vi "Vision Tracking Drive Control.vi"(11 "Cluster In":T11) -> (3 "Cluster Out":T11)   [LabVIEW 2018]
uses:
  <vilib>/Rock Robotics/WPI/MotorControl/WPI_MotorControlDeviceRef.ctl
  <vilib>/Rock Robotics/WPI/MotorControl/WPI_MotorControlType.ctl
  <vilib>/Rock Robotics/SystemInterfaces/DIO/FPGA_DIOPWMChannel.ctl
  <vilib>/Rock Robotics/WPI/PWM/WPI_PWMDeadband.ctl
  <vilib>/Rock Robotics/SystemInterfaces/DIO/FPGA_DIOChannel.ctl
  <vilib>/Rock Robotics/WPI/Joystick/WPI_JoystickDevRef.ctl
  <vilib>/Rock Robotics/WPI/Joystick/WPI_JoystickDeviceEnum.ctl
  <vilib>/Rock Robotics/WPI/DriverStation/WPI_DriverStationRobotMode2.ctl
  <vilib>/Rock Robotics/WPI/RobotDrive/WPI_RobotDriveDevRef.ctl
  Vision States.ctl
  <vilib>/Rock Robotics/WPI/ThirdParty/Phoenix-LabVIEW/Motor Controller/Controls/CTRE_Phoenix_MotorControl_ControlMode.ctl
  <vilib>/Rock Robotics/Network Tables/NT Read Number.vi
  Robot Global Data.vi
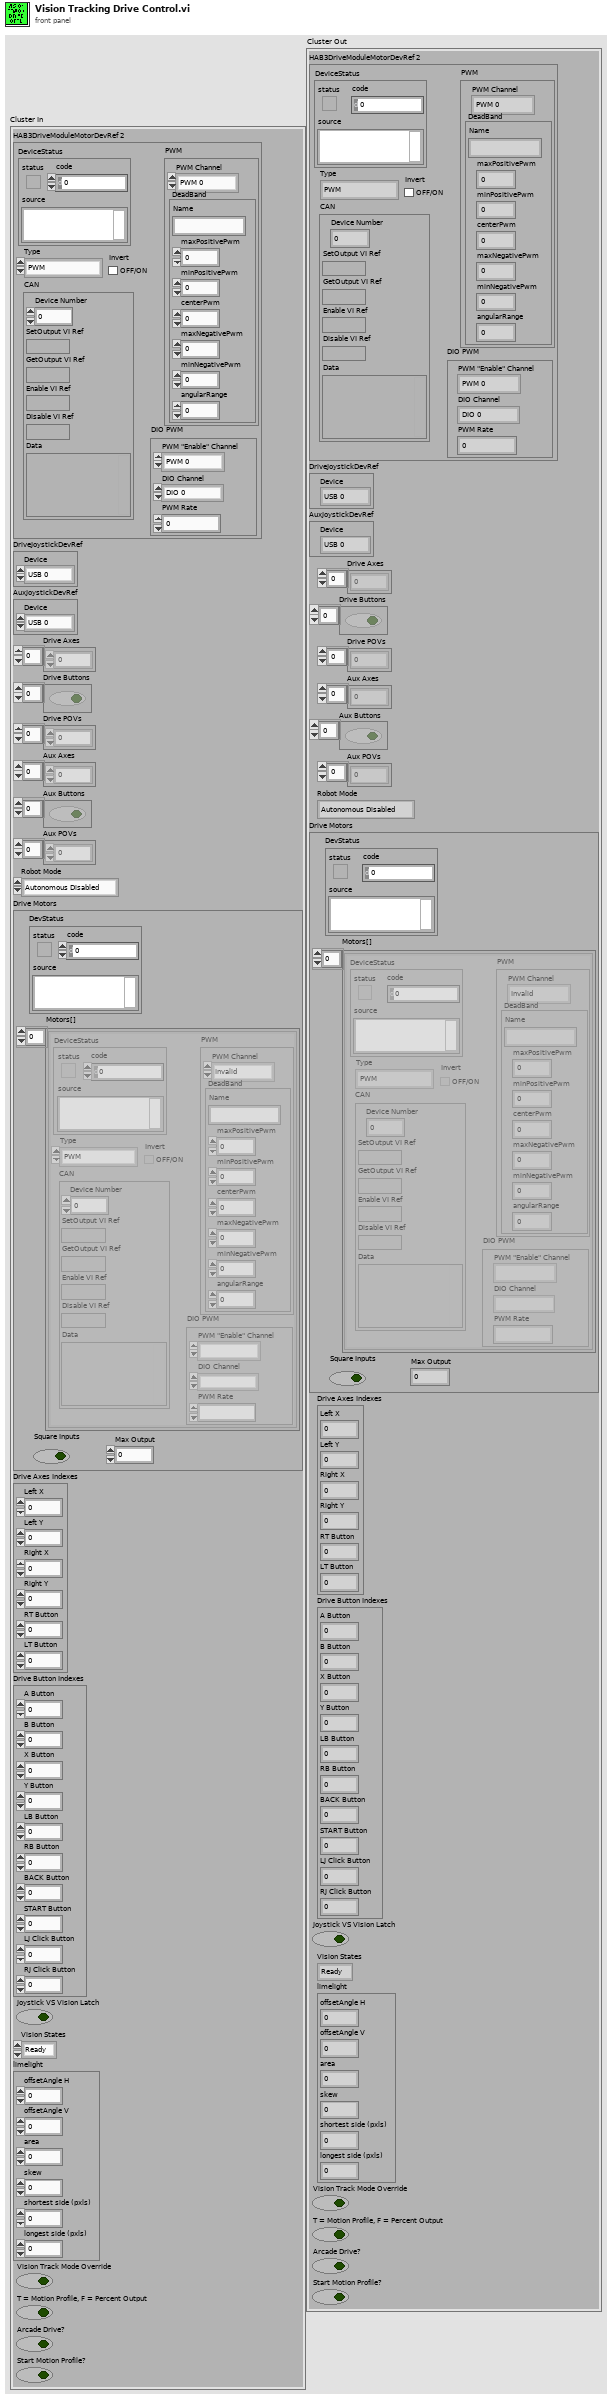
[diagram p1: front panel]
types:
  T1 = typedef "WPI_MotorControlDeviceRef.ctl" = cluster{"DeviceStatus":errorcluster, "Type":T2, "PWM":cluster{"PWM Channel":T3, "DeadBand":T4}, "CAN":cluster{"Device Number":u8, "SetOutput VI Ref":variant, "GetOutput VI Ref":variant, "Enable VI Ref":variant, "Disable VI Ref":variant, "Data":variant}, "Invert":bool, "DIO PWM":cluster{"PWM \"Enable\" Channel":T3, "DIOChannel":T5, "PWM Rate":dbl}}
  T2 = typedef "WPI_MotorControlType.ctl" = enum16{"PWM", "CAN", "DIO PWM"}
  T3 = typedef "FPGA_DIOPWMChannel.ctl" = enum8{"PWM 0", "PWM 1", "PWM 2", "PWM 3", "PWM 4", "PWM 5", "PWM 6", "PWM 7", "PWM 8", "PWM 9", "PWM MXP 0", "PWM MXP 1", "PWM MXP 2", "PWM MXP 3", "PWM MXP 4", "PWM MXP 5", "PWM MXP 6", "PWM MXP 7", "PWM MXP 8", "PWM MXP 9", "Invalid"}
  T4 = typedef "WPI_PWMDeadband.ctl" = cluster{"Name":string, "maxPositivePwm":i32, "minPositivePwm":i32, "centerPwm":i32, "maxNegativePwm":i32, "minNegativePwm":i32, "angularRange":u16}
  T5 = typedef "FPGA_DIOChannel.ctl" = enum8{"DIO 0", "DIO 1", "DIO 2", "DIO 3", "DIO 4", "DIO 5", "DIO 6", "DIO 7", "DIO 8", "DIO 9", "DIO MXP 0", "DIO MXP 1", "DIO MXP 2", "DIO MXP 3", "DIO MXP 4", "DIO MXP 5", "DIO MXP 6", "DIO MXP 7", "DIO MXP 8", "DIO MXP 9", "DIO MXP 10", "DIO MXP 11", "DIO MXP 12", "DIO MXP 13", "DIO MXP 14", "DIO MXP 15", "SPI Port CS1", "SPI Port CS2", "SPI Port CS3", "SPI Port MISO", "SPI Port MOSI", "Invalid"}
  T6 = typedef "WPI_JoystickDevRef.ctl" = cluster{"Device":T7}
  T7 = typedef "WPI_JoystickDeviceEnum.ctl" = enum16{"USB 0", "USB 1", "USB 2", "USB 3", "USB 4", "USB 5"}
  T8 = typedef "WPI_DriverStationRobotMode2.ctl" = enum16{"Autonomous Disabled", "Autonomous Enabled", "Teleop Disabled", "Teleop Enabled", "Disconnected", "Finish", "Test Disabled", "Test Enabled", "Emergency Stopped"}
  T9 = typedef "WPI_RobotDriveDevRef.ctl" = cluster{"DevStatus":errorcluster, "Motors[]":T1[], "Square Inputs":bool, "Max Output":dbl}
  T10 = typedef "Vision States.ctl" = enum16{"Ready", "Forward Until Target at Edge", "Vision Track"}
  T11 = cluster{"HAB3DriveModuleMotorDevRef 2":T1, "DriveJoystickDevRef":T6, "AuxJoystickDevRef":T6, "Drive Axes":dbl[], "Drive Buttons":bool[], "Drive POVs":i16[], "Aux Axes":dbl[], "Aux Buttons":bool[], "Aux POVs":i16[], "Robot Mode":T8, "Drive Motors":T9, "Drive Axes Indexes":cluster{"Left X":i32, "Left Y":i32, "Right X":i32, "Right Y":i32, "RT Button":i32, "LT Button":i32}, "Drive Button Indexes":cluster{"A Button":i32, "B Button":i32, "X Button":i32, "Y Button":i32, "LB Button":i32, "RB Button":i32, "BACK Button":i32, "START Button":i32, "LJ Click Button":i32, "RJ Click Button":i32}, "Joystick VS Vision Latch":bool, "Vision States":T10, "limelight":cluster{"offsetAngle H":dbl, "offsetAngle V":dbl, "area":dbl, "skew":dbl, "shortest side (pxls)":dbl, "longest side (pxls)":dbl}, "Vision Track Mode Override":bool, "T = Motion Profile, F = Percent Output":bool, "Arcade Drive?":bool, "Start Motion Profile?":bool}
  T12 = typedef "Which Robot Enum.ctl" = enum16{"Competition Bot", "Practice Bot", "Code Bot"}
  T13 = typedef "CTRE_Phoenix_MotorControl_ControlMode.ctl" = u16
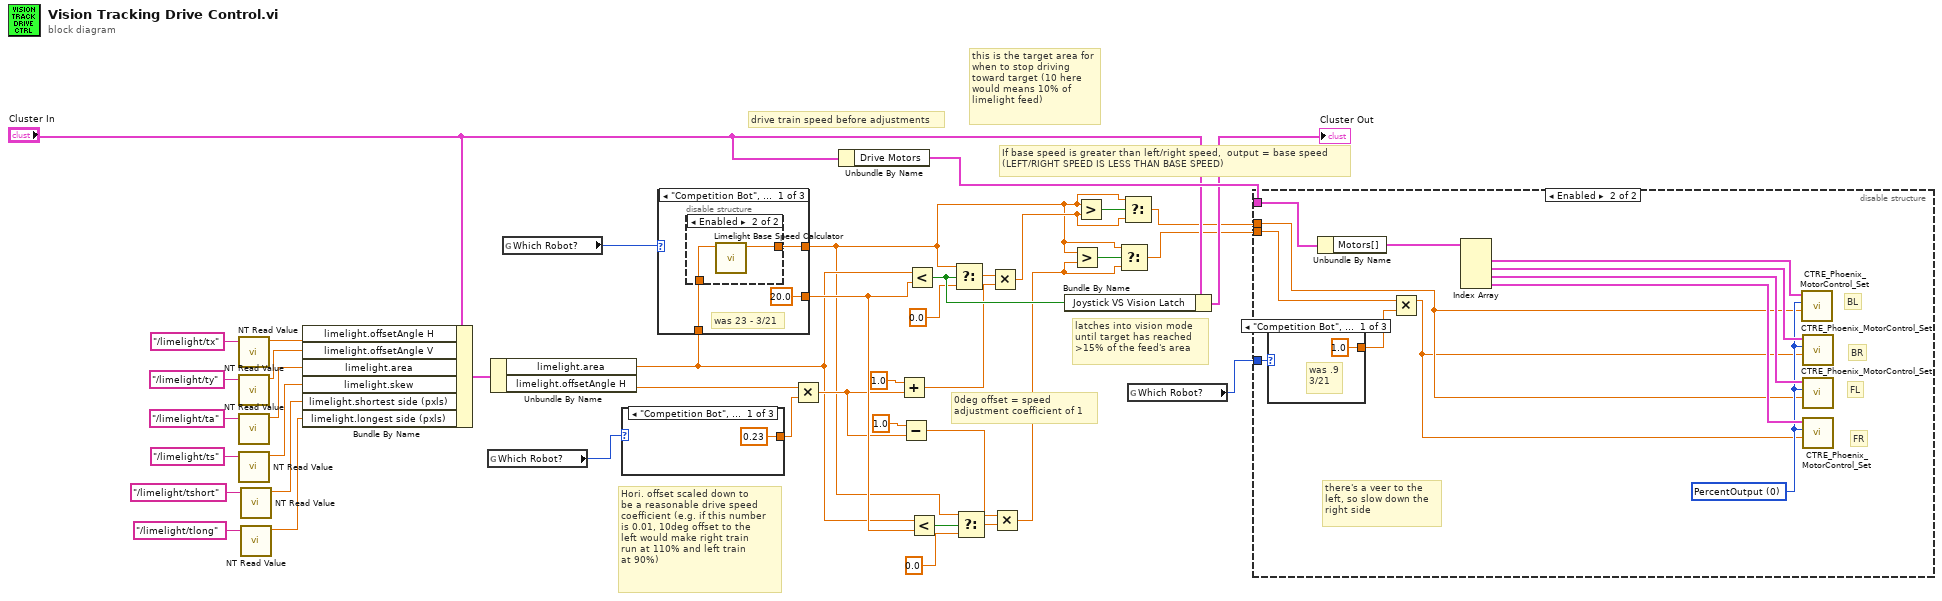
[diagram p0: block diagram]
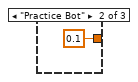
[diagram p2: hidden frame]
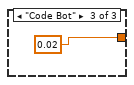
[diagram p3: hidden frame]
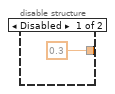
[diagram p4: hidden frame]
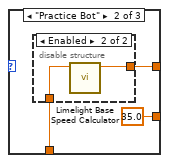
[diagram p5: hidden frame]
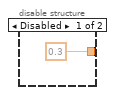
[diagram p6: hidden frame]
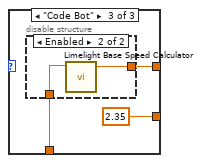
[diagram p7: hidden frame]
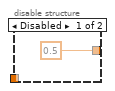
[diagram p8: hidden frame]
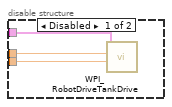
[diagram p9: hidden frame]
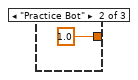
[diagram p10: hidden frame]
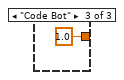
[diagram p11: hidden frame]
diagram:
  # "If base speed is greater than left/right speed,  output = base speed\n(LEFT/RIGHT SPEED IS LESS THAN BASE SPEED)"
  # "latches into vision mode \nuntil target has reached \n>15% of the feed's area"
  # "drive train speed before adjustments"
  # "this is the target area for\nwhen to stop driving \ntoward target (10 here \nwould means 10% of \nlimelight feed)"
  # "Hori. offset scaled down to\nbe a reasonable drive speed\ncoefficient (e.g. if this number\nis 0.01, 10deg offset to the \nleft would make right train \nrun at 110% and left train \nat 90%)"
  # "0deg offset = speed \nadjustment coefficient of 1"
  n1 = call-poly <vilib>:"NT Read Value.vi"("Name"="/limelight/tx") -> ("Numeric"=w18:dbl)  [unwired: 9 in, 1 out]
  n2 = call-poly <vilib>:"NT Read Value.vi"("Name"="/limelight/ty") -> ("Numeric"=w19:dbl)  [unwired: 9 in, 1 out]
  n3 = call-poly <vilib>:"NT Read Value.vi"("Name"="/limelight/ta") -> ("Numeric"=w20:dbl)  [unwired: 9 in, 1 out]
  n4 = call-poly <vilib>:"NT Read Value.vi"("Name"="/limelight/ts") -> ("Numeric"=w21:dbl)  [unwired: 9 in, 1 out]
  n5 = call-poly <vilib>:"NT Read Value.vi"("Name"="/limelight/tshort") -> ("Numeric"=w40:dbl)  [unwired: 9 in, 1 out]
  n6 = call-poly <vilib>:"NT Read Value.vi"("Name"="/limelight/tlong") -> ("Numeric"=w41:dbl)  [unwired: 9 in, 1 out]
  n7 = Bundle By Name(cluster="Cluster In", "limelight.offsetAngle H"=w18, "limelight.offsetAngle V"=w19, "limelight.area"=w20, "limelight.skew"=w21, "limelight.shortest side (pxls)"=w40, "limelight.longest side (pxls)"=w41) -> (w22:T11)
  n8 = global read "Robot Global Data.vi" "Which Robot?"() -> (w12:T12)
  n9 = Unbundle By Name(w22) -> ("limelight.area"=w8:dbl, "limelight.offsetAngle H"=w25:dbl)
  n10 = global read "Robot Global Data.vi" "Which Robot?"() -> (w13:T12)
  n11 = case shown="\"Competition Bot\", Default" w12 {
    tunnel: [0.23 ("y") 0.1 ("y") 0.02 ("y")] -> w26
    frame "Competition Bot", Default {
    }
    frame "Practice Bot" {
    }
    frame "Code Bot" {
    }
  }
  n12 = case shown="\"Competition Bot\", Default" w13 {
    tunnel: [20.0 35.0 2.35] -> w35
    tunnel: [w47 w53 w58] -> w4
    tunnel: w8 -> [w45 w51 w57]
    frame "Competition Bot", Default {
      # "was 23 - 3/21"
      n13 = disable-structure shown="Enabled" {
        disable-tunnel: [0.3 ("t") w49] -> w47
        disable-tunnel: w45 -> [_ w50]
        frame Disabled {
        }
        frame Enabled {
          n14 = call "Limelight Base Speed Calculator.vi"("Limelight TA"=w50) -> ("Base Drive Speed"=w49:dbl)  [unwired: 10 in]
        }
      }
    }
    frame "Practice Bot" {
      n15 = disable-structure shown="Enabled" {
        disable-tunnel: [0.3 ("t") w55] -> w53
        disable-tunnel: w51 -> [_ w56]
        frame Disabled {
        }
        frame Enabled {
          n16 = call "Limelight Base Speed Calculator.vi"("Limelight TA"=w56) -> ("Base Drive Speed"=w55:dbl)  [unwired: 10 in]
        }
      }
    }
    frame "Code Bot" {
      n17 = disable-structure shown="Enabled" {
        disable-tunnel: [0.5 ("t") w62] -> w58
        disable-tunnel: w57 -> [_ w61]
        frame Disabled {
        }
        frame Enabled {
          n18 = call "Limelight Base Speed Calculator.vi"("Limelight TA"=w61) -> ("Base Drive Speed"=w62:dbl)  [unwired: 10 in]
        }
      }
    }
  }
  n19 = Multiply(x=w25, y=w26) -> (x*y=w33:dbl)
  n20 = Unbundle By Name("Cluster In") -> ("Drive Motors"=w36:T9)
  n21 = Add(x=1.0, y=w33) -> (x+y=w29:dbl)
  n22 = Subtract(x=1.0, y=w33) -> (x-y=w34:dbl)
  n23 = Less?(x=w8, y=w35) -> (x < y?=w37:bool)
  n24 = Less?(x=w8, y=w35) -> (x < y?=w28:bool)
  n25 = Select(t=w4, s=w37, f=0.0) -> (s? t:f=w24:dbl)
  n26 = Select(t=w4, s=w28, f=0.0) -> (s? t:f=w31:dbl)
  n27 = Multiply(x=w24, y=w29) -> (x*y=w6:dbl)
  n28 = Multiply(x=w34, y=w31) -> (x*y=w3:dbl)
  n29 = Bundle By Name(cluster="Cluster In", "Joystick VS Vision Latch"=w37) -> (→"Cluster Out":T11)
  n30 = Greater?(x=w4, y=w3) -> (0:w5:bool)
  n31 = Greater?(x=w4, y=w6) -> (0:w7:bool)
  n32 = Select(t=w4, s=w5, f=w3) -> (s? t:f=w1:dbl)
  n33 = Select(t=w4, s=w7, f=w6) -> (s? t:f=w2:dbl)
  n34 = global read "Robot Global Data.vi" "Which Robot?"() -> (w11:T12)
  n35 = disable-structure shown="Enabled" {
    disable-tunnel: w36 -> [w65 w71]
    disable-tunnel: w1 -> [w64 w69]
    disable-tunnel: w2 -> [w63 w70]
    disable-tunnel: w11 -> [_ w66]
    frame Disabled {
      n36 = call <vilib>:"WPI_RobotDriveTankDrive.vi"("Right axis value"=w64, "Left axis value"=w63, "RobotDriveDevRef"=w65) -> ()  [unwired: 6 in, 3 out]
    }
    frame Enabled {
      w72 = T13 0 items=["PercentOutput"=0, "Position"=1, "Velocity"=2, "Current"=3, "Follower"=5, "MotionProfile"=6, "MotionMagic"=7, "MotionProfileArc"=10, "Disabled"=15] ("Control Mode")
      # "there's a veer to the\nleft, so slow down the\nright side"
      # "FR"
      # "FL"
      # "BR"
      # "BL"
      n37 = case shown="\"Competition Bot\", Default" w66 {
        tunnel: [1.0 ("y") 1.0 ("y") 1.0 ("y")] -> w67
        frame "Competition Bot", Default {
          # "was .9\n3/21"
        }
        frame "Practice Bot" {
        }
        frame "Code Bot" {
        }
      }
      n38 = Unbundle By Name(w71) -> ("Motors[]"=w77:T1[])
      n39 = Multiply(x=w69, y=w67) -> (x*y=w68:dbl)
      n40 = Index Array(array=w77) -> (element #1=w76:T1, element #2=w73:T1, element #3=w75:T1, element #4=w74:T1)  [unwired: 4 in]
      n41 = call <vilib>:"CTRE_Phoenix_MotorControl_Set.vi"("Output"=w70, "Control Mode"=w72, "PhoenixMotorControlDevRef"=w76) -> ()  [unwired: 7 in, 2 out]
      n42 = call <vilib>:"CTRE_Phoenix_MotorControl_Set.vi"("Output"=w68, "Control Mode"=w72, "PhoenixMotorControlDevRef"=w73) -> ()  [unwired: 7 in, 2 out]
      n43 = call <vilib>:"CTRE_Phoenix_MotorControl_Set.vi"("Output"=w70, "Control Mode"=w72, "PhoenixMotorControlDevRef"=w75) -> ()  [unwired: 7 in, 2 out]
      n44 = call <vilib>:"CTRE_Phoenix_MotorControl_Set.vi"("Output"=w68, "Control Mode"=w72, "PhoenixMotorControlDevRef"=w74) -> ()  [unwired: 7 in, 2 out]
    }
  }
